vi "Write K_I.vi"(8 "error in (no error)":errorcluster, 10 "Real Matrix":T1, 11 "PID Controller in":refnum<class "PID Controller.lvclass">) -> (0 "error out":errorcluster, 3 "PID Controller out":refnum<class "PID Controller.lvclass">)   [LabVIEW 2014, in "Controller Library.lvlib" / "PID Controller.lvclass"]
uses:
  PID Controller.lvclass
  <vilib>/Analysis/Matrix/Datatypes/RealMatrix.ctl
  PID Controller.lvclass/PID Controller.ctl
  <vilib>/Analysis/Matrix/NI_Matrix.lvlib
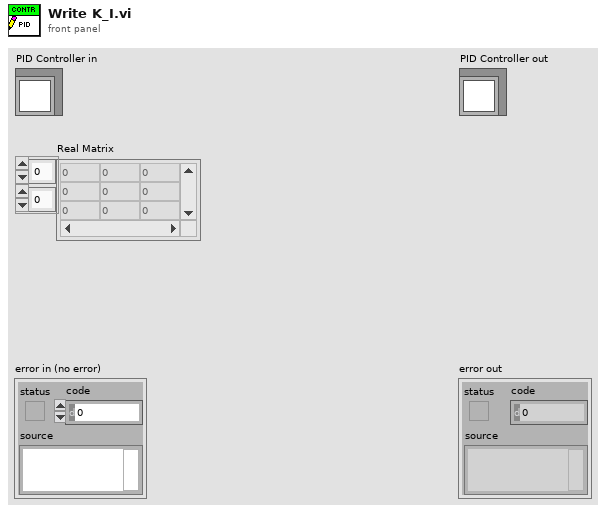
[diagram p1: front panel]
types:
  T1 = typedef "NI_Matrix.lvlib/RealMatrix.ctl" = dbl[][]
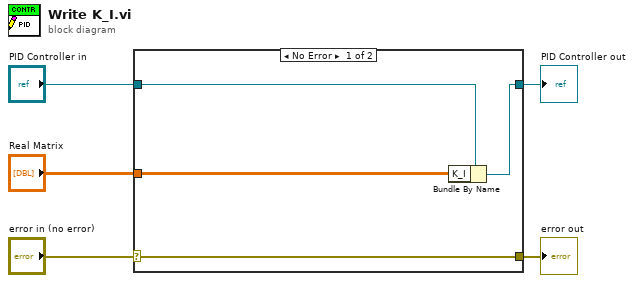
[diagram p0: block diagram]
diagram:
  n1 = case shown="No Error" "error in (no error)" {
    selector: "error in (no error)" -> [w9 w10]
    tunnel: [w9 w10] -> w4
    tunnel: [w7 w11] -> w2
    tunnel: "PID Controller in" -> [w8 w11]
    tunnel: "Real Matrix" -> [w6 _]
    frame No Error {
      n2 = Bundle By Name(cluster=w8, "K_I"=w6) -> (w7:refnum<class "PID Controller.lvclass">)
    }
    frame Error {
    }
  }
  "error out" <- w4
  "PID Controller out" <- w2
